vi "Run Server.vi"(8 "error in (no error)":errorcluster, 11 "Stop OOB Server UE":refnum<user-event>) -> (0 "error out":errorcluster)   [LabVIEW 2025, in "Automotive-Vision-OOBService_server.lvlib"]
uses:
  Automotive-Vision-OOBService_server.lvlib
  <vilib>/gRPC/LabVIEW gRPC Servicer/ServiceBase/ServiceBase.lvclass
  <vilib>/gRPC/LabVIEW gRPC Servicer/Servicer/Servicer.lvclass
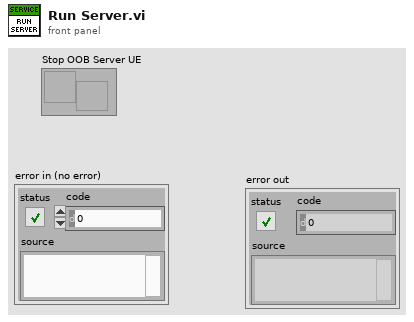
[diagram p1: front panel]
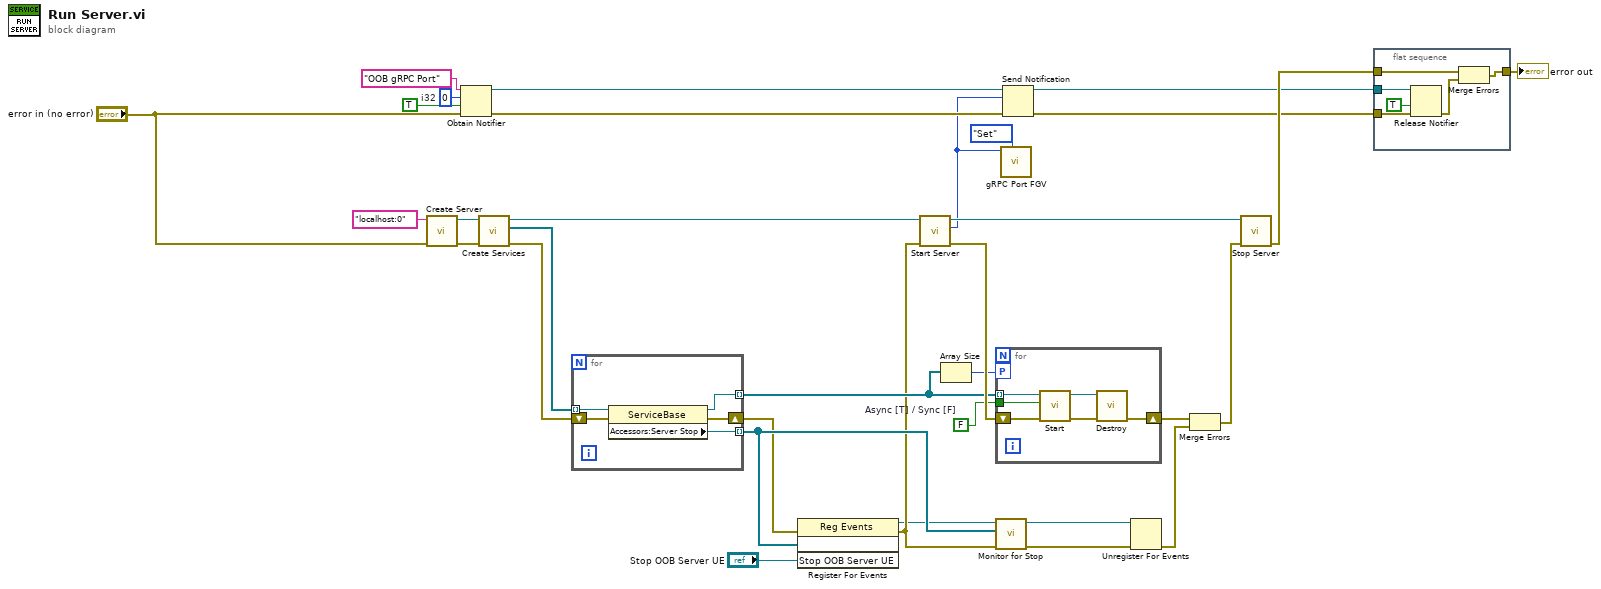
[diagram p0: block diagram]
diagram:
  w29 = FALSE  # Async [T] / Sync [F]
  w14 = 0  # i32
  n1 = call <vilib>:"Create Server.vi"("error in"="error in (no error)", "Server Address"="localhost:0") -> ("error out"=w17:errorcluster, "gRPC server out"=w32:refnum<class "Servicer.lvclass">)  [unwired: 8 in]
  n2 = Obtain Notifier(name (unnamed)="OOB gRPC Port", notification data type=w14, create if not found? (T)=TRUE, error in (no error)="error in (no error)") -> (notifier out=w12:refnum<notifier>, error out=w8:errorcluster)  [unwired: 1 out]
  n3 = call "Create Services.vi"("error in (no error)"=w17, "gRPC server in"=w32) -> ("error out"=w16:errorcluster, "gRPC services out"=w15:refnum<class "ServiceBase.lvclass">[], "gRPC server out"=w31:refnum<class "Servicer.lvclass">)  [unwired: 7 in]
  n4 = for {
    tunnel: [w37] -> w26 mode=indexing
    shift-right: [w36] -> w25
    shift-left: w16 -> [w34]
    tunnel: [w38] -> w27 mode=indexing
    tunnel: w15 -> [w35] mode=indexing
    n5 = property class="ServiceBase"(reference=w35, error in=w34) -> (reference out=w38:refnum<class "ServiceBase.lvclass">, error out=w36:errorcluster, "Accessors:Server Stop"=w37:refnum<user-event>)
  }
  n6 = register-events(error in=w25, w26, "Stop OOB Server UE") -> (reference out=w1:refnum<event-registration>, error out=w24:errorcluster)  [unwired: 1 in]
  n7 = call <vilib>:"Start Server.vi"("error in"=w24, "gRPC server in"=w31) -> ("error out"=w30:errorcluster, "Listening Port"=w3:i32, "gRPC server out"=w33:refnum<class "Servicer.lvclass">)  [unwired: 7 in]
  n8 = Array Size(array=w27) -> (size(s)=w28:i32)
  n9 = for {
    tunnel: w27 -> [w42] mode=indexing
    tunnel: w29 -> [w40]
    workers-P: w28 -> [_]
    shift-right: [w39] -> w23
    shift-left: w30 -> [w41]
    n10 = call-dynamic "Start.vi"("error in"=w41, "ASync [T]"=w40, "gRPC service in"=w42) -> ("error out"=w43:errorcluster, "gRPC service out"=w44:refnum<class "ServiceBase.lvclass">)  [unwired: 7 in]
    n11 = call-dynamic "Destroy.vi"("error in"=w43, "gRPC service in"=w44) -> ("error out"=w39:errorcluster)  [unwired: 8 in, 1 out]
  }
  n12 = call "Monitor for Stop.vi"("error in (no error)"=w24, "service stop events"=w26, "Event Registration Refnum in"=w1) -> ("error out"=w19:errorcluster, "Event Registration Refnum out"=w21:refnum<event-registration>)  [unwired: 7 in]
  n13 = call "gRPC Port FGV.vi"("Op (Get)"=enum16{"Get", "Set"}."Set", "Listening Port in"=w3) -> ()  [unwired: 9 in, 1 out]
  n14 = Send Notification(notification=w3, notifier=w12, error in (no error)=w8) -> (notifier out=w11:refnum<notifier>, error out=w9:errorcluster)
  n15 = Unregister For Events(event registration refnum=w21, error in=w19) -> (error out=w20:errorcluster)
  n16 = Merge Errors(w23, w20) -> (w22:errorcluster)
  n17 = call <vilib>:"Stop Server.vi"("error in"=w22, "gRPC server in"=w33) -> ("error out"=w18:errorcluster)  [unwired: 9 in]
  n18 = flat-sequence {
    tunnel: w11 -> [w50]
    tunnel: w18 -> [w48]
    tunnel: [w47] -> w10
    tunnel: w9 -> [w45]
    frame #0 {
      n19 = Release Notifier(notifier=w50, force destroy? (F)=TRUE, error in (no error)=w45) -> (error out=w46:errorcluster)  [unwired: 2 out]
      n20 = Merge Errors(w48, w46) -> (w47:errorcluster)
    }
  }
  "error out" <- w10
